vi "TEST MMI Scaling (Alternatives).vi"() -> ()   [LabVIEW 2013, in "IObject.lvclass"]
uses:
  IObject.lvclass
  IContainer/Interaction/Interaction.lvclass
  IContainer/Viewport/Viewport.lvclass
  IContainer/Divider/Splitter/Splitter.lvclass
  IContainer/Alternative/Alternative.lvclass
  Object/Object.lvclass
panel:
  out "XY Graph 5":cluster{"X":dbl, "Y":dbl}[](graph)
  in  "XY Button 0":bool
  out "XY Graph 3":cluster{"X":dbl, "Y":dbl}[](graph)
  in  "XY Button 2":bool
  out "XY Graph 1":cluster{"X":dbl, "Y":dbl}[](graph)
  in  "XY Button 4":bool
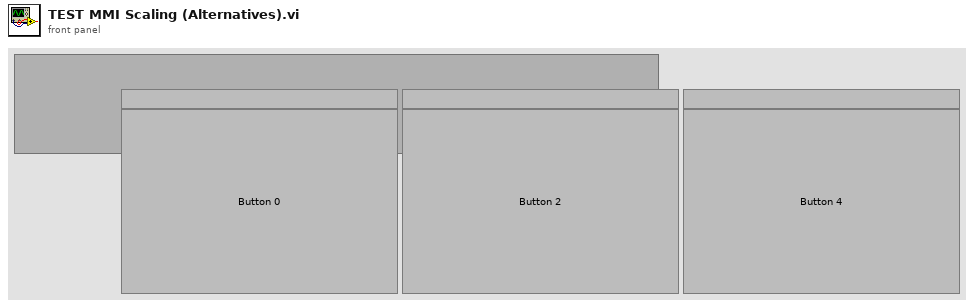
[diagram p1: front panel]
types:
  T1 = cluster{"Left":dbl, "Top":dbl, "Right":dbl, "Bottom":dbl}
  T2 = typedef "LVRectTypeDef.ctl" = cluster{"Left":i16, "Top":i16, "Right":i16, "Bottom":i16}
  T3 = typedef "LVPoint32TypeDef.ctl" = cluster{"Horizontal":i32, "Vertical":i32}
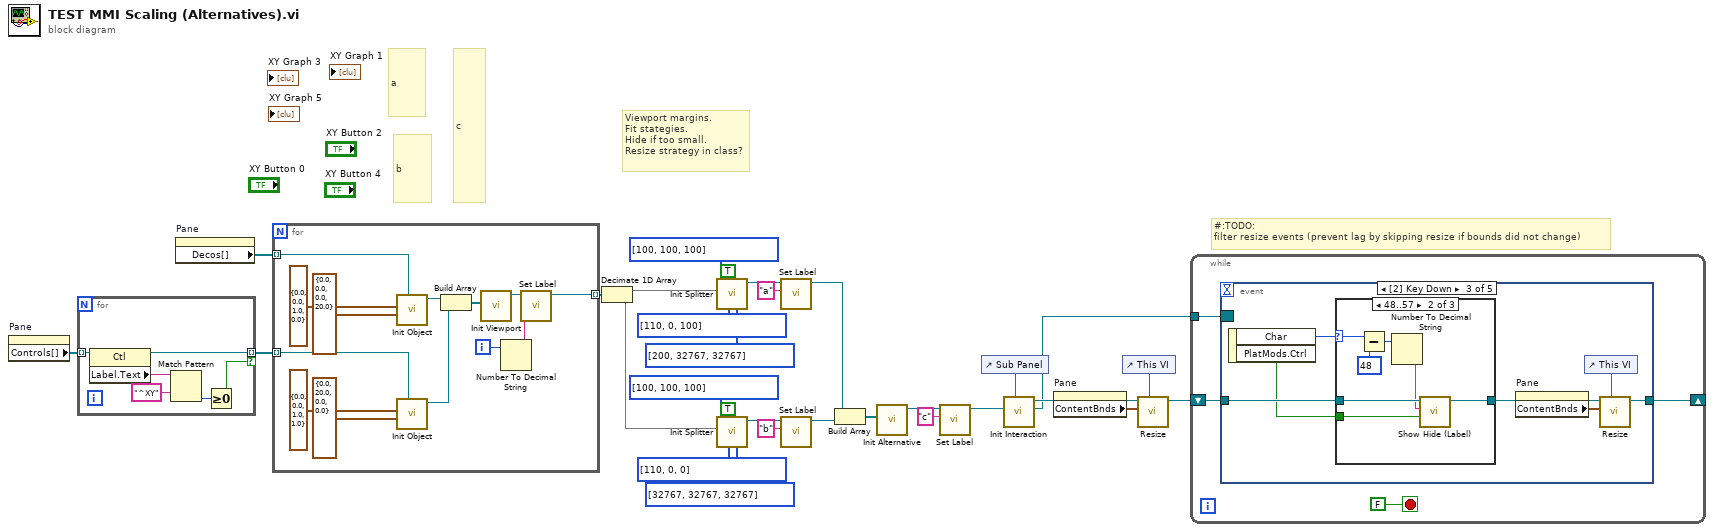
[diagram p0: block diagram]
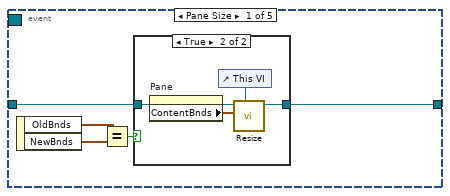
[diagram p2: hidden frame]
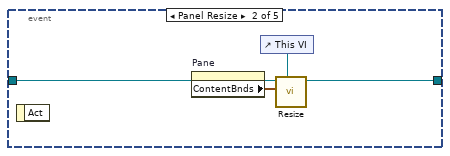
[diagram p4: hidden frame]
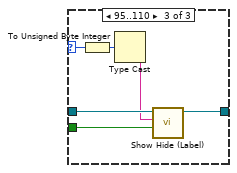
[diagram p6: hidden frame]
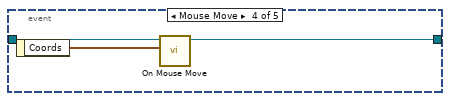
[diagram p7: hidden frame]
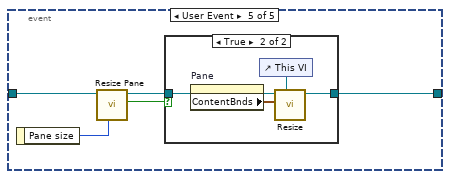
[diagram p8: hidden frame]
diagram:
  # "c"
  # "b"
  # "a"
  # "#:TODO:\nfilter resize events (prevent lag by skipping resize if bounds did not change)"
  # "Viewport margins.\nFit stategies.\nHide if too small.\nResize strategy in class?"
  n1 = property on="Pane" class="Pane"() -> ("Controls[]"=w11:refnum<vi>[])  [unwired: 2 in, 2 out]
  n2 = for {
    tunnel: w11 -> [w31] mode=indexing
    tunnel: [w34] -> w10 mode=indexing if=w32
    n3 = property class="Ctl"(reference=w31) -> (reference out=w34:refnum<vi>, "Label.Text"=w36:string)  [unwired: 1 in, 1 out]
    n4 = Match Pattern(string=w36, regular expression="^XY") -> (offset past match=w33:i32)  [unwired: 1 in, 3 out]
    n5 = Greater Or Equal To 0?(x=w33) -> (x >= 0?=w32:bool)
  }
  n6 = property on="Pane" class="Pane"() -> ("Decos[]"=w28:refnum<vi>[])  [unwired: 2 in, 2 out]
  n7 = for {
    tunnel: w28 -> [w49] mode=indexing
    tunnel: [w38] -> w22 mode=indexing
    tunnel: w10 -> [w42] mode=indexing
    i -> [w48]
    n8 = call "Init Object.vi"("GObj Refnum"=w49, "B [0, 0, 0, 0]"=T1 {"Left"=0.0, "Top"=0.0, "Right"=0.0, "Bottom"=20.0} ("B"), "A [0, 0, 1, 1]"=T1 {"Left"=0.0, "Top"=0.0, "Right"=1.0, "Bottom"=0.0} ("A")) -> ("MMI Scaling out"=w40:refnum<class "Object.lvclass">)  [unwired: 7 in, 1 out]
    n9 = call "Init Object.vi"("GObj Refnum"=w42, "B [0, 0, 0, 0]"=T1 {"Left"=0.0, "Top"=20.0, "Right"=0.0, "Bottom"=0.0} ("B"), "A [0, 0, 1, 1]"=T1 {"Left"=0.0, "Top"=0.0, "Right"=1.0, "Bottom"=1.0} ("A")) -> ("MMI Scaling out"=w39:refnum<class "Object.lvclass">)  [unwired: 7 in, 1 out]
    n10 = Build Array(w40, w39) -> (w45:refnum<class "Object.lvclass">[])
    n11 = call "Init Viewport.vi"("Items"=w45) -> ("Viewport out"=w37:refnum<class "Viewport.lvclass">)  [unwired: 9 in, 1 out]
    n12 = Number To Decimal String(number=w48) -> (decimal integer string=w41:string)  [unwired: 1 in]
    n13 = call "Set Label.vi"("Label"=w41, "MMI Scaling in"=w37) -> ("MMI Scaling out"=w38:refnum<class "Viewport.lvclass">)  [unwired: 8 in, 1 out]
  }
  n14 = Decimate 1D Array(w22) -> (w23:refnum<class "Viewport.lvclass">[], w15:refnum<class "Viewport.lvclass">[])
  n15 = call "Init Splitter.vi"("Maximal size"=i16[] [200, 32767, 32767] ("Minimal size"), "Minimal size"=i16[] [110, 0, 100], "Vertical? [F, hor.]"=TRUE, "Relative size"=i16[] [100, 100, 100] ("Minimal size"), "Items"=w23) -> ("Splitter out"=w30:refnum<class "Splitter.lvclass">)  [unwired: 5 in, 1 out]
  n16 = call "Init Splitter.vi"("Maximal size"=i16[] [32767, 32767, 32767] ("Minimal size"), "Minimal size"=i16[] [110, 0, 0], "Vertical? [F, hor.]"=TRUE, "Relative size"=i16[] [100, 100, 100] ("Minimal size"), "Items"=w15) -> ("Splitter out"=w16:refnum<class "Splitter.lvclass">)  [unwired: 5 in, 1 out]
  n17 = call "Set Label.vi"("Label"="a", "MMI Scaling in"=w30) -> ("MMI Scaling out"=w2:refnum<class "Splitter.lvclass">)  [unwired: 8 in, 1 out]
  n18 = call "Set Label.vi"("Label"="b", "MMI Scaling in"=w16) -> ("MMI Scaling out"=w4:refnum<class "Splitter.lvclass">)  [unwired: 8 in, 1 out]
  n19 = Build Array(w2, w4) -> (w14:refnum<class "Splitter.lvclass">[])
  n20 = call "Init Alternative.vi"("Items"=w14) -> ("Viewport out"=w12:refnum<class "Alternative.lvclass">)  [unwired: 9 in, 1 out]
  n21 = call "Set Label.vi"("Label"="c", "MMI Scaling in"=w12) -> ("MMI Scaling out"=w1:refnum<class "Alternative.lvclass">)  [unwired: 8 in, 1 out]
  n22 = control-ref of="Sub Panel"() -> (w3:refnum<vi>)
  n23 = call "Init Interaction.vi"("Sub Panel"=w3, "IObject"=w1) -> ("Interaction Splitter Resize"=w5:refnum<event-registration>, "Interaction out"=w7:refnum<class "Interaction.lvclass">)  [unwired: 6 in, 2 out]
  n24 = property on="Pane" class="Pane"() -> ("ContentBnds"=w8:T2)  [unwired: 2 in, 2 out]
  n25 = control-ref of="This VI"() -> (w9:refnum<vi>)
  n26 = call-dynamic "Resize.vi"("VI Refnum"=w9, "Bounds"=w8, "MMI Scaling in"=w7) -> ("MMI Scaling out"=w6:refnum<class "Interaction.lvclass">)  [unwired: 6 in, 2 out]
  n27 = while {
    shift-right: [w51] -> _
    shift-left: w6 -> [w53]
    tunnel: w5 -> [w50]
    stop <- FALSE stop-if-true
    n28 = event shown="[2] Key Down" {
      selector: w50 -> [_ _ _ _ _]
      dyn-events: _ -> [_ _ _ _ _]
      timeout: _ -> [_ _ _ _ _]
      tunnel: w53 -> [w58 w67 w69 w91 w96]
      tunnel: [w57 w66 w72 w89 w92] -> w51
      event Pane Size {
        n29 = event-data() -> ("OldBnds"=w56:T2, "NewBnds"=w55:T2)  [unwired: 1 in]
        n30 = Equal?(x=w56, y=w55) -> (x = y?=w54:bool)
        n31 = case shown="True" w54 {
          tunnel: w58 -> [w59 w63]
          tunnel: [w59 w60] -> w57
          frame False {
          }
          frame True {
            n32 = property on="Pane" class="Pane"() -> ("ContentBnds"=w62:T2)  [unwired: 2 in, 2 out]
            n33 = control-ref of="This VI"() -> (w61:refnum<vi>)
            n34 = call-dynamic "Resize.vi"("VI Refnum"=w61, "Bounds"=w62, "MMI Scaling in"=w63) -> ("MMI Scaling out"=w60:refnum<class "Interaction.lvclass">)  [unwired: 6 in, 2 out]
          }
        }
      }
      event Panel Resize {
        n35 = event-data() -> ()  [unwired: 1 in, 1 out]
        n36 = property on="Pane" class="Pane"() -> ("ContentBnds"=w65:T2)  [unwired: 2 in, 2 out]
        n37 = control-ref of="This VI"() -> (w64:refnum<vi>)
        n38 = call-dynamic "Resize.vi"("VI Refnum"=w64, "Bounds"=w65, "MMI Scaling in"=w67) -> ("MMI Scaling out"=w66:refnum<class "Interaction.lvclass">)  [unwired: 6 in, 2 out]
      }
      event Key Down {
        n39 = event-data() -> ("Char"=w71:i16, "PlatMods.Ctrl"=w68:bool)  [unwired: 1 in]
        n40 = case shown="48..57" w71 {
          selector: w71 -> [_ w82 w86]
          tunnel: [w75 w78 w87] -> w70
          tunnel: w69 -> [w75 w80 w88]
          tunnel: w68 -> [_ w77 w84]
          frame Default {
          }
          frame 48..57 {
            n41 = Subtract(x=w82, y=i16 48) -> (x-y=w79:i16)
            n42 = Number To Decimal String(number=w79) -> (decimal integer string=w76:string)  [unwired: 1 in]
            n43 = call-dynamic "Show Hide (Label).vi"("Show? [T]"=w77, "Label"=w76, "MMI Scaling in"=w80) -> ("MMI Scaling out"=w78:refnum<class "Interaction.lvclass">)  [unwired: 6 in, 2 out]
          }
          frame 95..110 {
            n44 = To Unsigned Byte Integer(number=w86) -> (unsigned 8bit integer=w85:u8)
            n45 = Type Cast(x=w85) -> (*(type *) &x=w83:string)  [unwired: 1 in]
            n46 = call-dynamic "Show Hide (Label).vi"("Show? [T]"=w84, "Label"=w83, "MMI Scaling in"=w88) -> ("MMI Scaling out"=w87:refnum<class "Interaction.lvclass">)  [unwired: 6 in, 2 out]
          }
        }
        n47 = property on="Pane" class="Pane"() -> ("ContentBnds"=w74:T2)  [unwired: 2 in, 2 out]
        n48 = control-ref of="This VI"() -> (w73:refnum<vi>)
        n49 = call-dynamic "Resize.vi"("VI Refnum"=w73, "Bounds"=w74, "MMI Scaling in"=w70) -> ("MMI Scaling out"=w72:refnum<class "Interaction.lvclass">)  [unwired: 6 in, 2 out]
      }
      event Mouse Move {
        n50 = event-data() -> ("Coords"=w90:T3)  [unwired: 1 in]
        n51 = call "On Mouse Move.vi"("Coords"=w90, "Interaction in"=w91) -> ("Interaction out"=w89:refnum<class "Interaction.lvclass">)  [unwired: 8 in, 1 out]
      }
      event User Event {
        n52 = event-data() -> ("Pane size"=w95:i32)  [unwired: 1 in]
        n53 = call-dynamic "Resize Pane.vi"("Pane size"=w95, "IContainer in"=w96) -> ("Resized?"=w94:bool, "IContainer out"=w93:refnum<class "Interaction.lvclass">)  [unwired: 7 in, 1 out]
        n54 = case shown="True" w94 {
          tunnel: [w97 w99] -> w92
          tunnel: w93 -> [w97 w98]
          frame False {
          }
          frame True {
            n55 = property on="Pane" class="Pane"() -> ("ContentBnds"=w101:T2)  [unwired: 2 in, 2 out]
            n56 = control-ref of="This VI"() -> (w100:refnum<vi>)
            n57 = call-dynamic "Resize.vi"("VI Refnum"=w100, "Bounds"=w101, "MMI Scaling in"=w98) -> ("MMI Scaling out"=w99:refnum<class "Interaction.lvclass">)  [unwired: 6 in, 2 out]
          }
        }
      }
    }
  }
